vi "Compute UC Tau Tick (g, s) & (dg, ds).vi"(8 "1/2 pi f":dbl[unit], 9 "Tick Length (0.01)":dbl=0.01, 10 "Tick Index":i32, 11 "tau_i":dbl[unit]) -> (0 "tau_i (ns)":dbl, 1 "label?":bool, 2 "Tick (dg, ds)":T1, 3 "Tick center (g, s)":T1, 4 "long tick?":bool)   [LabVIEW 2019]
uses:
  Phasor (g, s).ctl
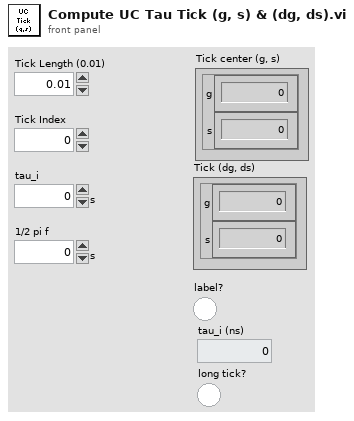
[diagram p1: front panel]
types:
  T1 = typedef "Phasor (g, s).ctl" = cluster{"g":dbl, "s":dbl}
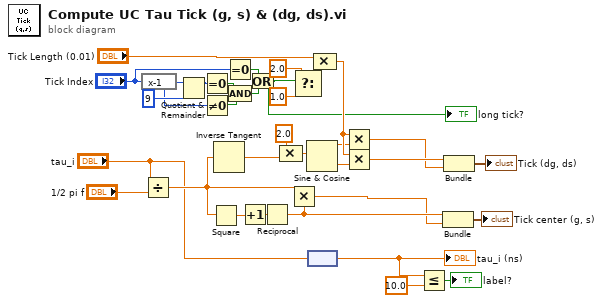
[diagram p0: block diagram]
diagram:
  n1 = expression code="x-1"("Tick Index") -> (w30:i32)
  n2 = Divide(x="tau_i", y="1/2 pi f") -> (x/y=w16:dbl)
  n3 = Quotient & Remainder(x=w30, y=9 ("# Decades")) -> (x-y*floor(x/y)=w23:i32)  [unwired: 1 out]
  n4 = Equal To 0?(x=w23) -> (x = 0?=w29:bool)
  n5 = Not Equal To 0?(x=w30) -> (x != 0?=w32:bool)
  n6 = Square(x=w16) -> (x^2=w14:dbl)
  n7 = Inverse Tangent(1:w16) -> (0:w13:dbl)
  n8 = Equal To 0?(x="Tick Index") -> (x = 0?=w28:bool)
  n9 = Compound Arithmetic op=AND(w29, w32) -> (w31:bool)
  n10 = Increment(x=w14) -> (x+1=w15:dbl)
  n11 = Or(x=w28, y=w31) -> (x .or. y?=w1:bool)
  "long tick?" <- w1
  n12 = Reciprocal(x=w15) -> (1/x=w8:dbl)
  n13 = Compound Arithmetic op=MULTIPLY(2.0 ("value"), w13) -> (w20:dbl)
  n14 = Multiply(x=w16, y=w8) -> (x*y=w7:dbl)
  n15 = Select(t=2.0 ("value"), s=w1, f=1.0) -> (s? t:f=w26:dbl)
  n16 = Sine & Cosine(0:w20) -> (1:w17:dbl, 2:w18:dbl)
  n17 = node("tau_i") -> (w4:dbl)
  "tau_i (ns)" <- w4
  n18 = Compound Arithmetic op=MULTIPLY("Tick Length (0.01)", w26) -> (w22:dbl)
  n19 = Multiply(x=w22, y=w17) -> (x*y=w10:dbl)
  n20 = Multiply(x=w22, y=w18) -> (x*y=w11:dbl)
  n21 = Less Or Equal?(x=w4, y=10.0) -> (x <= y?=→"label?":bool)
  n22 = Bundle(w8, w7) -> (→"Tick center (g, s)":cluster{dbl, dbl})  [unwired: 1 in]
  n23 = Bundle(w11, w10) -> (→"Tick (dg, ds)":cluster{dbl, dbl})  [unwired: 1 in]
